vi "Culab GEMM And Operations Float.vi"(11 "dimension size":i32=16384) -> (3 "Culab Time":dbl)   [LabVIEW 2020]
uses:
  <vilib>/Ngene/CuLab - GPU Accelerated Toolkit/Toolkit/Low_Level/Tensor_Classes/T_Children/T2D/Controls/T2D_Dims.ctl
  <vilib>/Ngene/CuLab - GPU Accelerated Toolkit/Toolkit/Low_Level/Tensor_Classes/T_Children/T2D/T2D_Children/T2D_SGL/Create.vi
  <vilib>/Ngene/CuLab - GPU Accelerated Toolkit/Toolkit/Low_Level/Tensor_Classes/T_Children/T2D/T2D_Children/T2D_SGL/Create_Push.vi
  <vilib>/Ngene/CuLab - GPU Accelerated Toolkit/Toolkit/Low_Level/Tensor_Classes/T_Children/T0D/T0D_Children/T0D_SGL/Create.vi
  <vilib>/Ngene/CuLab - GPU Accelerated Toolkit/Toolkit/API/Linear Algebra/BLAS3/gemm/CU_gemm/CU_Sgemm.vi
  <vilib>/Ngene/CuLab - GPU Accelerated Toolkit/Toolkit/API/Numeric/Absolute/T2D/CU_Absolute_T2D_SGL.vi
  <vilib>/Ngene/CuLab - GPU Accelerated Toolkit/Toolkit/API/Numeric/Add/T2D/CU_AddC_T2D_SGL.vi
  <vilib>/Ngene/CuLab - GPU Accelerated Toolkit/Toolkit/API/Elementary/Exponential/Natural Logarithm/T2D/CU_Natural_Logarithm_T2D_SGL.vi
  <vilib>/Ngene/CuLab - GPU Accelerated Toolkit/Toolkit/API/Array/Array Max Min/T2D/CU_Array_Max_Min_T2D_SGL.vi
  <vilib>/Ngene/CuLab - GPU Accelerated Toolkit/Toolkit/Low_Level/Tensor_Classes/T_Children/T0D/T0D_Children/T0D_SGL/Pull.vi
  <vilib>/Ngene/CuLab - GPU Accelerated Toolkit/Toolkit/CuLab.lvlib
  <vilib>/Ngene/CuLab - GPU Accelerated Toolkit/Toolkit/Low_Level/Tensor_Classes/T_Children/T2D/T2D_Children/T2D_SGL/T2D_SGL.lvclass
  <vilib>/Ngene/CuLab - GPU Accelerated Toolkit/Toolkit/Low_Level/Tensor_Classes/T_Children/T0D/T0D_Children/T0D_SGL/T0D_SGL.lvclass
  <vilib>/Analysis/NI_AALBase.lvlib
panel:
  out "max value":dbl
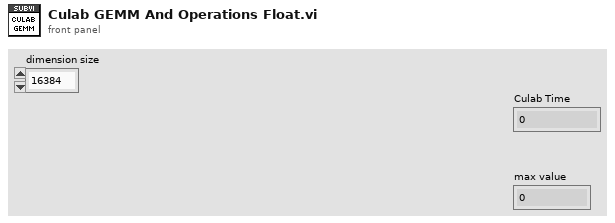
[diagram p1: front panel]
types:
  T1 = typedef "CuLab.lvlib/T2D_Dims.ctl" = cluster{"H":i32, "W":i32}
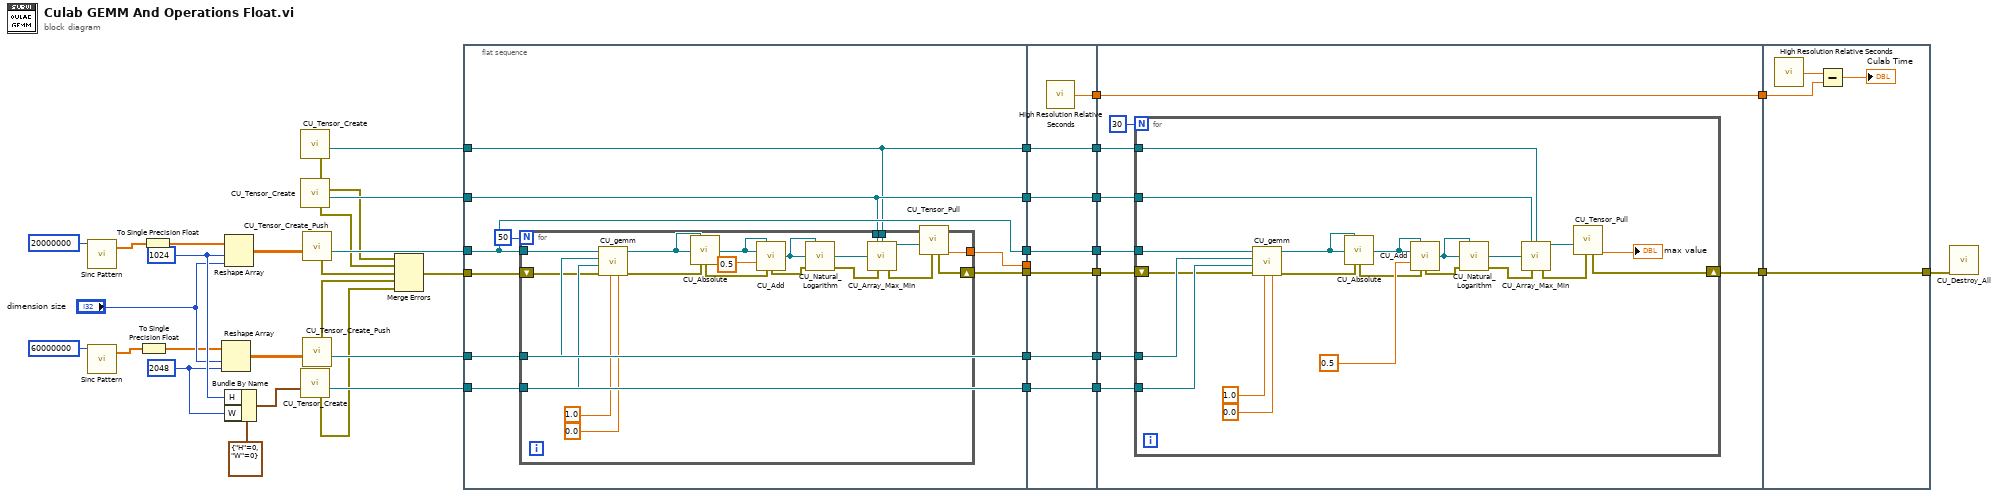
[diagram p0: block diagram]
diagram:
  w23 = 2048 ("dimension size")
  w24 = 1024 ("dimension size")
  n1 = call <vilib>:"Sinc Pattern.vi"("samples"=20000000) -> ("Sinc Pattern"=w31:dbl[])  [unwired: 3 in, 1 out]
  n2 = call <vilib>:"Sinc Pattern.vi"("samples"=60000000) -> ("Sinc Pattern"=w30:dbl[])  [unwired: 3 in, 1 out]
  n3 = To Single Precision Float(number=w30) -> (single precision float=w15:sgl[])
  n4 = To Single Precision Float(number=w31) -> (single precision float=w16:sgl[])
  n5 = Reshape Array(w15, "dimension size", w23) -> (w18:sgl[][])
  n6 = Reshape Array(w16, w24, "dimension size") -> (w19:sgl[][])
  n7 = Bundle By Name(cluster=T1 {"H"=0, "W"=0} ("T2D_Dims"), "H"=w24, "W"=w23) -> (w25:T1)
  n8 = call-poly <vilib>:"CU_Tensor_Create.vi"() -> ("T0D_SGL out"=w22:refnum<class "T0D_SGL.lvclass">, "error out"=w1:errorcluster)  [unwired: 10 in]
  n9 = call-poly <vilib>:"CU_Tensor_Create.vi"() -> ("T0D_SGL out"=w21:refnum<class "T0D_SGL.lvclass">, "error out"=w2:errorcluster)  [unwired: 10 in]
  n10 = call-poly <vilib>:"CU_Tensor_Create.vi"("T2D_Dims"=w25) -> ("T2D_SGL out"=w27:refnum<class "T2D_SGL.lvclass">, "error out"=w4:errorcluster)  [unwired: 9 in]
  n11 = call-poly <vilib>:"CU_Tensor_Create_Push.vi"("CPU_Data_2D_SGL"=w19) -> ("T2D_SGL out"=w29:refnum<class "T2D_SGL.lvclass">, "error out"=w6:errorcluster)  [unwired: 9 in]
  n12 = call-poly <vilib>:"CU_Tensor_Create_Push.vi"("CPU_Data_2D_SGL"=w18) -> ("T2D_SGL out"=w28:refnum<class "T2D_SGL.lvclass">, "error out"=w3:errorcluster)  [unwired: 9 in]
  n13 = Merge Errors(w1, w2, w6, w3, w4) -> (w5:errorcluster)
  n14 = flat-sequence {
    tunnel: w21 -> [w46]
    tunnel: w22 -> [w45]
    tunnel: w27 -> [w49]
    tunnel: w28 -> [w50]
    tunnel: w29 -> [w47]
    tunnel: [w50] -> w14
    tunnel: [w49] -> w13
    tunnel: [w45] -> w12
    tunnel: [w46] -> w11
    tunnel: [w48] -> w10
    tunnel: [w47] -> w9
    tunnel: [w43] -> w7
    tunnel: w5 -> [w42]
    tunnel: [w78] -> w41
    tunnel: [w77] -> w40
    tunnel: [w76] -> w39
    tunnel: [w75] -> w38
    tunnel: [w74] -> w37
    tunnel: [w73] -> w36
    tunnel: w14 -> [w76]
    tunnel: w13 -> [w75]
    tunnel: w12 -> [w74]
    tunnel: w11 -> [w73]
    tunnel: w10 -> [_]
    tunnel: w9 -> [w77]
    tunnel: [w72] -> w8
    tunnel: w7 -> [w72]
    tunnel: w41 -> [w87]
    tunnel: [w87] -> w35
    tunnel: w40 -> [w86]
    tunnel: w39 -> [w85]
    tunnel: w38 -> [w84]
    tunnel: w37 -> [w83]
    tunnel: w36 -> [w82]
    tunnel: [w81] -> w34
    tunnel: w8 -> [w79]
    tunnel: w35 -> [w111]
    tunnel: w34 -> [w109]
    tunnel: [w109] -> w20
    frame #0 {
      n15 = for {
        N: 50 -> [_]
        tunnel: w50 -> [w61]
        tunnel: w49 -> [w60]
        tunnel: [w59] -> w48
        tunnel: w47 -> [w58]
        tunnel: w46 -> [w54]
        tunnel: w45 -> [w53]
        shift-right: [w52] -> w43
        shift-left: w42 -> [w51]
        n16 = call-poly <vilib>:"CU_gemm.vi"("beta"=sgl 0.0, "alpha"=sgl 1.0, "error in (no error)"=w51, "C"=w60, "B"=w61, "A"=w58) -> ("error out"=w67:errorcluster, "C out"=w69:refnum<class "T2D_SGL.lvclass">)  [unwired: 4 in]
        n17 = call-poly <vilib>:"CU_Absolute.vi"("Dest in"=w69, "x"=w69, "error in (no error)"=w67) -> ("Dest out"=w68:refnum<class "T2D_SGL.lvclass">, "error out"=w66:errorcluster)  [unwired: 11 in]
        n18 = call-poly <vilib>:"CU_Add.vi"("Dest in"=w68, "x"=w68, "y"=sgl 0.5, "error in (no error)"=w66) -> ("Dest out"=w70:refnum<class "T2D_SGL.lvclass">, "error out"=w65:errorcluster)  [unwired: 10 in]
        n19 = call-poly <vilib>:"CU_Natural_Logarithm.vi"("Dest in"=w70, "x"=w70, "error in (no error)"=w65) -> ("ln(x)"=w71:refnum<class "T2D_SGL.lvclass">, "error out"=w64:errorcluster)  [unwired: 11 in]
        n20 = call-poly <vilib>:"CU_Array_Max_Min.vi"("Min Dest in"=w54, "Max Dest in"=w53, "Tensor in"=w71, "error in (no error)"=w64) -> ("Max Dest out"=w62:refnum<class "T0D_SGL.lvclass">, "error out"=w63:errorcluster)  [unwired: 7 in, 3 out]
        n21 = call-poly <vilib>:"CU_Tensor_Pull.vi"("error in (no error)"=w63, "T0D_SGL in"=w62) -> ("Dest out"=w59:sgl, "error out"=w52:errorcluster)  [unwired: 7 in, 1 out]
      }
    }
    frame #1 {
      n22 = call <vilib>:"High Resolution Relative Seconds.vi"() -> ("relative seconds"=w78:dbl)
    }
    frame #2 {
      n23 = for {
        N: 30 -> [_]
        tunnel: w86 -> [w108]
        tunnel: w85 -> [w107]
        tunnel: w84 -> [w96]
        tunnel: w83 -> [w91]
        tunnel: w82 -> [w90]
        shift-right: [w89] -> w81
        shift-left: w79 -> [w88]
        n24 = call-poly <vilib>:"CU_gemm.vi"("beta"=0.0, "alpha"=1.0, "error in (no error)"=w88, "C"=w96, "B"=w107, "A"=w108) -> ("error out"=w99:errorcluster, "C out"=w94:refnum<class "T2D_SGL.lvclass">)  [unwired: 4 in]
        n25 = call-poly <vilib>:"CU_Absolute.vi"("Dest in"=w94, "x"=w94, "error in (no error)"=w99) -> ("Dest out"=w95:refnum<class "T2D_SGL.lvclass">, "error out"=w100:errorcluster)  [unwired: 11 in]
        n26 = call-poly <vilib>:"CU_Add.vi"("Dest in"=w95, "x"=w95, "y"=sgl 0.5, "error in (no error)"=w100) -> ("Dest out"=w93:refnum<class "T2D_SGL.lvclass">, "error out"=w101:errorcluster)  [unwired: 10 in]
        n27 = call-poly <vilib>:"CU_Natural_Logarithm.vi"("Dest in"=w93, "x"=w93, "error in (no error)"=w101) -> ("ln(x)"=w92:refnum<class "T2D_SGL.lvclass">, "error out"=w102:errorcluster)  [unwired: 11 in]
        n28 = call-poly <vilib>:"CU_Array_Max_Min.vi"("Min Dest in"=w90, "Max Dest in"=w91, "Tensor in"=w92, "error in (no error)"=w102) -> ("Max Dest out"=w105:refnum<class "T0D_SGL.lvclass">, "error out"=w103:errorcluster)  [unwired: 7 in, 3 out]
        n29 = call-poly <vilib>:"CU_Tensor_Pull.vi"("error in (no error)"=w103, "T0D_SGL in"=w105) -> ("Dest out"=→"max value":sgl, "error out"=w89:errorcluster)  [unwired: 7 in, 1 out]
      }
    }
    frame #3 {
      n30 = call <vilib>:"High Resolution Relative Seconds.vi"() -> ("relative seconds"=w112:dbl)
      n31 = Subtract(x=w112, y=w111) -> (x-y=→"Culab Time":dbl)
    }
  }
  n32 = call <vilib>:"CU_Destroy_All.vi"("error in"=w20) -> ()  [unwired: 10 in, 1 out]
